vi "GenerateFilePaths.vi"(1 "Logfile? (F)":bool, 2 "DAQmx (F)":bool, 3 "Extension (.tdms)":string=".tdms", 4 "Device Name":string="Sensors_DAQ1") -> (0 "Path":path=path "C:/Labview Test Data/2018-08-08/Sensors_DAQ1_Log.tdms")   [LabVIEW 2018]
uses:
  Global Variables.vi
  <vilib>/Utility/file.llb/Read Delimited Spreadsheet (string).vi
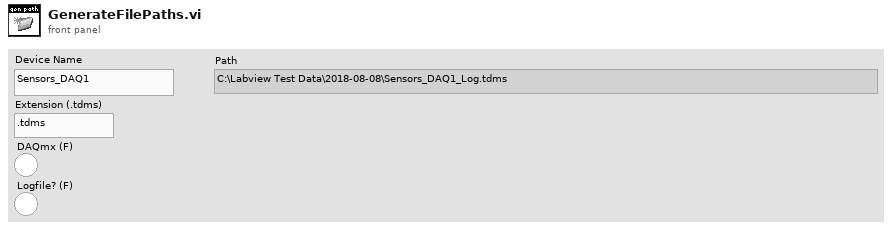
[diagram p1: front panel]
types:
  T1 = cluster{"Project":u16, "SubFolder":string, "Filename (Meas. Description)":string, "Measurement index":i32}
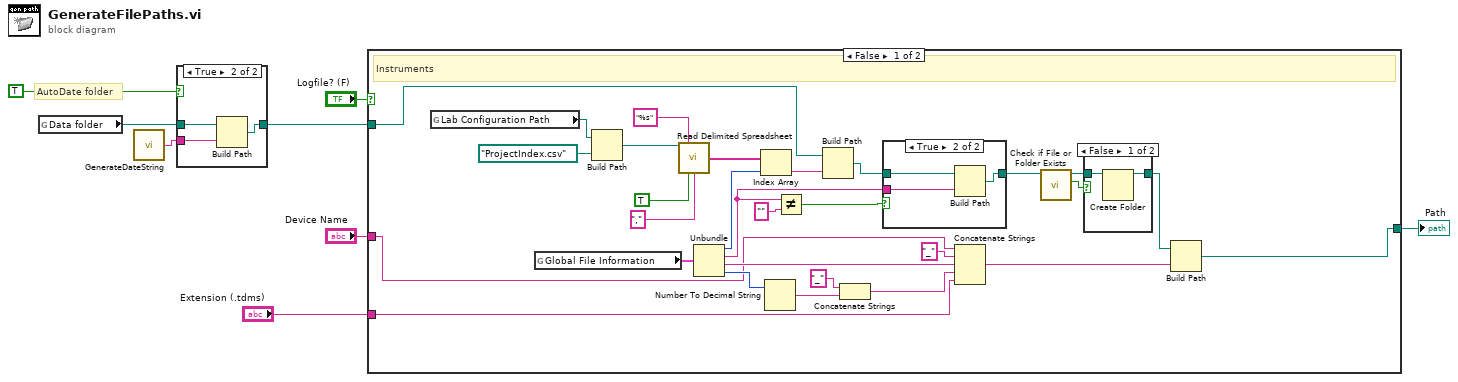
[diagram p0: block diagram]
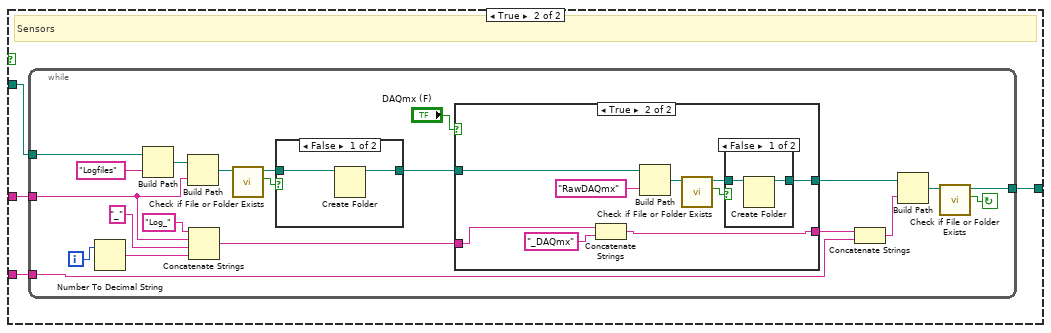
[diagram p4: hidden frame]
diagram:
  # "AutoDate folder"
  n1 = global read "Global Variables.vi" "Data folder"() -> (w6:path)
  n2 = call "GenerateDateString.vi"() -> ("String"=w8:string)
  n3 = case shown="True" TRUE ("Auto Date folder") {
    tunnel: w6 -> [w9 w12]
    tunnel: [w9 w10] -> w4
    tunnel: w8 -> [_ w11]
    frame False {
    }
    frame True {
      n4 = Build Path(base path=w12, name or relative path=w11) -> (appended path=w10:path)
    }
  }
  n5 = case shown="False" "Logfile? (F)" {
    tunnel: w4 -> [w19 w52]
    tunnel: "Device Name" -> [w18 w51]
    tunnel: "Extension (.tdms)" -> [w17 w50]
    tunnel: [w16 w49] -> w1
    frame False {
      # "Instruments"
      n6 = global read "Global Variables.vi" "Lab Configuration Path"() -> (w36:path)
      n7 = global read "Global Variables.vi" "Global File Information"() -> (w41:T1)
      n8 = Build Path(base path=w36, name or relative path=path "ProjectIndex.csv" ("vi path")) -> (appended path=w37:path)
      n9 = call-poly <vilib>:"Read Delimited Spreadsheet.vi"("file path (dialog if empty)"=w37, "format (%s)"="%s", "transpose? (F)"=TRUE, "delimiter (\\t)"="," ("delimiter (\\t)")) -> ("first row"=w35:string[])  [unwired: 6 in, 5 out]
      n10 = Unbundle(w41) -> ("Project"=w34:u16, "SubFolder"=w24:string, "Filename (Meas. Description)"=w30:string, "Measurement index"=w29:i32)
      n11 = Index Array(array=w35, index=w34) -> (element=w33:string)
      n12 = Number To Decimal String(number=w29) -> (decimal integer string=w14:string)  [unwired: 1 in]
      n13 = Not Equal?(x=w24, y="") -> (x != y?=w25:bool)
      n14 = Build Path(base path=w19, name or relative path=w33) -> (appended path=w32:path)
      n15 = Concatenate Strings("_" ("element"), w14) -> (w28:string)
      n16 = case shown="True" w25 {
        tunnel: w32 -> [w45 w48]
        tunnel: [w45 w47] -> w22
        tunnel: w24 -> [_ w46]
        frame False {
        }
        frame True {
          n17 = Build Path(base path=w48, name or relative path=w46) -> (appended path=w47:path)
        }
      }
      n18 = Concatenate Strings(w18, "_" ("string"), w30, w28, w17) -> (w27:string)
      n19 = call <vilib>:"Check if File or Folder Exists.vi"("path"=w22) -> ("file or folder exists?"=w20:bool, "dup path"=w23:path)  [unwired: 8 in, 1 out]
      n20 = case shown="False" w20 {
        tunnel: w23 -> [w43 w44]
        tunnel: [w42 w44] -> w21
        frame False {
          n21 = Create Folder(path (use dialog)=w43) -> (created path=w42:path)  [unwired: 2 in, 2 out]
        }
        frame True {
        }
      }
      n22 = Build Path(base path=w21, name or relative path=w27) -> (appended path=w16:path)
    }
    frame True {
      # "Sensors"
      n23 = while {
        tunnel: w51 -> [w61]
        tunnel: w50 -> [w56]
        tunnel: w52 -> [w62]
        tunnel: [w53] -> w49
        i -> [w58]
        stop <- w59 continue-if-true
        n24 = Number To Decimal String(number=w58) -> (decimal integer string=w66:string)  [unwired: 1 in]
        n25 = Build Path(base path=w62, name or relative path="Logfiles") -> (appended path=w73:path)
        n26 = Build Path(base path=w73, name or relative path=w61) -> (appended path=w68:path)
        n27 = Concatenate Strings("Log_" ("string"), w61, "_" ("string"), w66) -> (w72:string)
        n28 = call <vilib>:"Check if File or Folder Exists.vi"("path"=w68) -> ("file or folder exists?"=w69:bool, "dup path"=w67:path)  [unwired: 8 in, 1 out]
        n29 = case shown="False" w69 {
          tunnel: w67 -> [w89 w90]
          tunnel: [w88 w90] -> w70
          frame False {
            n30 = Create Folder(path (use dialog)=w89) -> (created path=w88:path)  [unwired: 2 in, 2 out]
          }
          frame True {
          }
        }
        n31 = case shown="True" "DAQmx (F)" {
          tunnel: [w74 w83] -> w55
          tunnel: w72 -> [w74 w82]
          tunnel: [w75 w81] -> w71
          tunnel: w70 -> [w75 w78]
          frame False {
          }
          frame True {
            n32 = Concatenate Strings(w82, "_DAQmx" ("string")) -> (w83:string)
            n33 = Build Path(base path=w78, name or relative path="RawDAQmx") -> (appended path=w79:path)
            n34 = call <vilib>:"Check if File or Folder Exists.vi"("path"=w79) -> ("file or folder exists?"=w84:bool, "dup path"=w80:path)  [unwired: 8 in, 1 out]
            n35 = case shown="False" w84 {
              tunnel: w80 -> [w86 w87]
              tunnel: [w85 w87] -> w81
              frame False {
                n36 = Create Folder(path (use dialog)=w86) -> (created path=w85:path)  [unwired: 2 in, 2 out]
              }
              frame True {
              }
            }
          }
        }
        n37 = Concatenate Strings(w55, w56) -> (w54:string)
        n38 = Build Path(base path=w71, name or relative path=w54) -> (appended path=w60:path)
        n39 = call <vilib>:"Check if File or Folder Exists.vi"("path"=w60) -> ("file or folder exists?"=w59:bool, "dup path"=w53:path)  [unwired: 8 in, 1 out]
      }
    }
  }
  "Path" <- w1
